vi "Init Rx - UDP Connection.vi"(8 "error in (no error)":errorcluster, 11 "Rx Loop Data in":T1) -> (0 "error out":errorcluster, 3 "Rx Loop Data out":T1)   [LabVIEW 2019, in "UDP-Custom-Device Engine.lvlib"]
uses:
  UDP-Custom-Device Engine.lvlib
  Types/Engine - Rx Loop Data.ctl
  <vilib>/NI VeriStand/VeriStand Data/Byte Buffer/Byte Buffer.lvclass
  Types/Engine - General Resources.ctl
  <vilib>/NI VeriStand/VeriStand Data/Typedefs/Typedefs.Data Types.ctl
  Shared/Types/Shared - Duplex Settings.ctl
  Shared/Types/Shared - Header Details.ctl
  Types/Engine - Data Conversion Config.ctl
  <vilib>/NI VeriStand/VeriStand Data/Byte Buffer/Byte Buffer.Mapping.ctl
  Types/Engine - Rx Runtime Resources.ctl
  Types/Engine - Execution Config.ctl
  Shared/Types/Shared - Thread Management.ctl
  Types/Engine - Rx New Data Options Support.ctl
  Shared/Types/Shared - New Data Options.ctl
  Types/Engine - Rx Channel Refs.ctl
  <vilib>/NI/NIVS Inline Async API/_Data Access Engine/Data Access Engine/Types/Write.DVR.ctl
  <vilib>/NI/NIVS Inline Async API/_Data Access Engine/Access Type Classes/Write/Write.lvclass
  Types/Engine - Debug Resources.ctl
  <vilib>/Utility/tcp.llb/UDP Multicast Read-Only Open.vi
  <vilib>/NI/NIVS Inline Async API/_Data Access Engine/Data Access Engine/Data Access Engine.lvclass
  <vilib>/NI VeriStand/VeriStand Data/VeriStand Data.lvlib
  Shared/UDP-Custom-Device Shared.lvlib
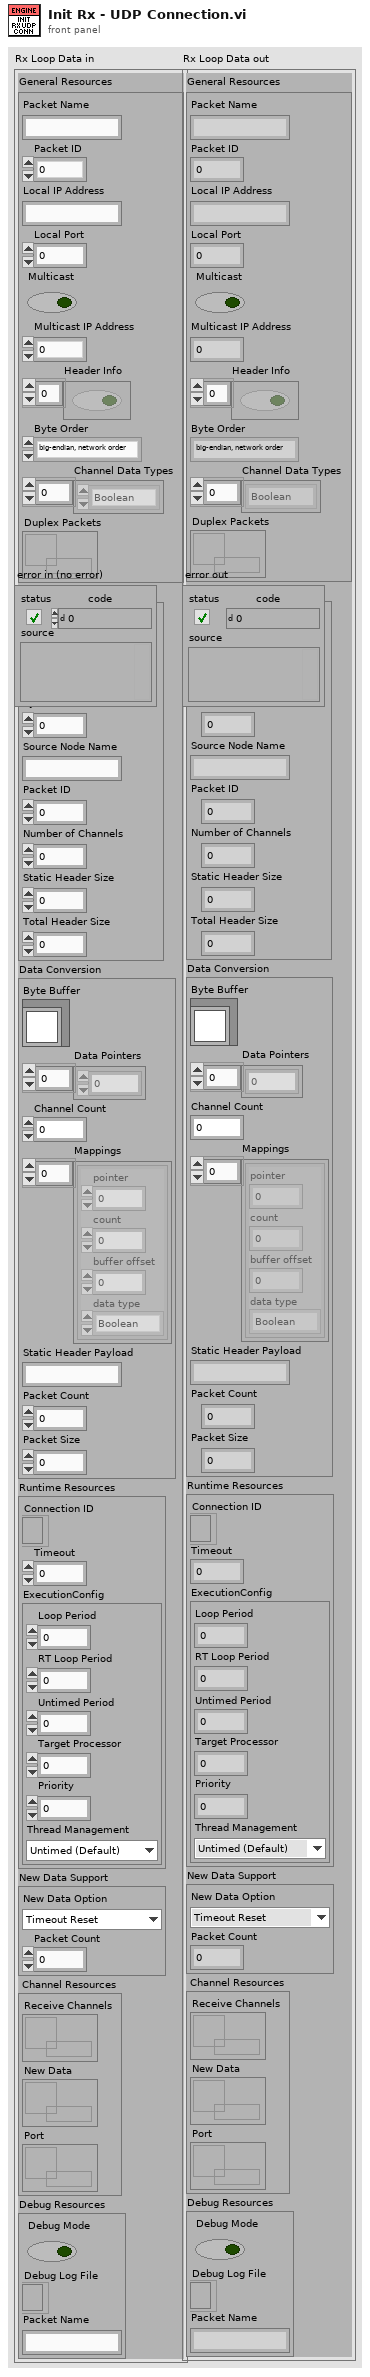
[diagram p1: front panel]
types:
  T1 = typedef "UDP-Custom-Device Engine.lvlib/Engine - Rx Loop Data.ctl" = cluster{"General Resources":T2, "Header Details":T4, "Data Conversion":T5, "Runtime Resources":T7, "New Data Support":T10, "Channel Resources":T12, "Debug Resources":T14}
  T2 = typedef "UDP-Custom-Device Engine.lvlib/Engine - General Resources.ctl" = cluster{"Packet Name":string, "Packet ID":i32, "Local IP Address":string, "Local Port":i32, "Multicast":bool, "Multicast IP Address":u32, "Header Info":bool[], "Byte Order":enum16{"big-endian, network order", "native, host order", "little-endian"}, "Channel Data Types":T3[], "Duplex Packets":refnum<data-value>}
  T3 = typedef "VeriStand Data.lvlib/Typedefs.Data Types.ctl" = enum16{"Boolean", "Single", "Double", "I8", "I16", "I32", "I64", "U8", "U16", "U32", "U64"}
  T4 = typedef "UDP-Custom-Device Shared.lvlib/Shared - Header Details.ctl" = cluster{"Packet Size":u16, "Protocol Revision":u8, "System Definition Version":u64, "Source Node Name":string, "Packet ID":u32, "Number of Channels":u32, "Static Header Size":u16, "Total Header Size":u16}
  T5 = typedef "UDP-Custom-Device Engine.lvlib/Engine - Data Conversion Config.ctl" = cluster{"Byte Buffer":refnum<class "Byte Buffer.lvclass">, "Data Pointers":u64[], "Channel Count":i32, "Mappings":T6[], "Static Header Payload":string, "Packet Count":dbl, "Packet Size":i32}
  T6 = typedef "VeriStand Data.lvlib/Byte Buffer.lvclass/Byte Buffer.Mapping.ctl" = cluster{"pointer":u64, "count":i64, "buffer offset":u64, "data type":T3}
  T7 = typedef "UDP-Custom-Device Engine.lvlib/Engine - Rx Runtime Resources.ctl" = cluster{"Connection ID":refnum<k16>, "Timeout":i32, "ExecutionConfig":T8}
  T8 = typedef "UDP-Custom-Device Engine.lvlib/Engine - Execution Config.ctl" = cluster{"Loop Period":i64, "RT Loop Period":i64, "Untimed Period":u32, "Target Processor":i32, "Priority":i32, "Thread Management":T9}
  T9 = typedef "UDP-Custom-Device Shared.lvlib/Shared - Thread Management.ctl" = enum16{"Untimed (Default)", "Timed (High Priority)"}
  T10 = typedef "UDP-Custom-Device Engine.lvlib/Engine - Rx New Data Options Support.ctl" = cluster{"New Data Option":T11, "Packet Count":dbl}
  T11 = typedef "UDP-Custom-Device Shared.lvlib/Shared - New Data Options.ctl" = enum16{"Timeout Reset", "Counter"}
  T12 = typedef "UDP-Custom-Device Engine.lvlib/Engine - Rx Channel Refs.ctl" = cluster{"Receive Channels":T13, "New Data":T13, "Port":T13}
  T13 = typedef "Data Access Engine.lvlib/Data Access Engine.lvclass/Write.DVR.ctl" = refnum<data-value>
  T14 = typedef "UDP-Custom-Device Engine.lvlib/Engine - Debug Resources.ctl" = cluster{"Debug Mode":bool, "Debug Log File":refnum<file>, "Packet Name":string}
  T15 = typedef "UDP-Custom-Device Shared.lvlib/Shared - Duplex Settings.ctl" = cluster{"Transmit Packet ID":i32, "Receive Packet ID":i32, "Multicast":bool, "Multicast Address":string, "IP Address":string, "Port":u16, "TTL":u16, "Duplex Connection":refnum<k16>}
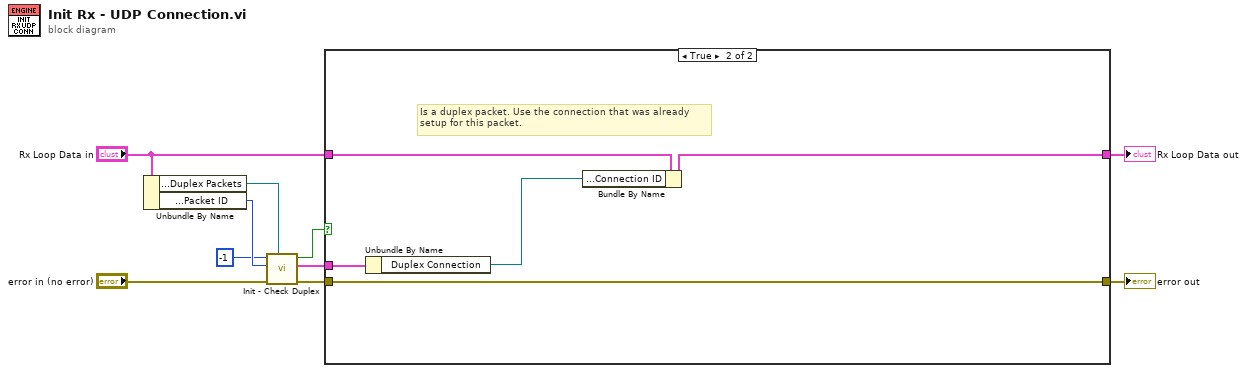
[diagram p0: block diagram]
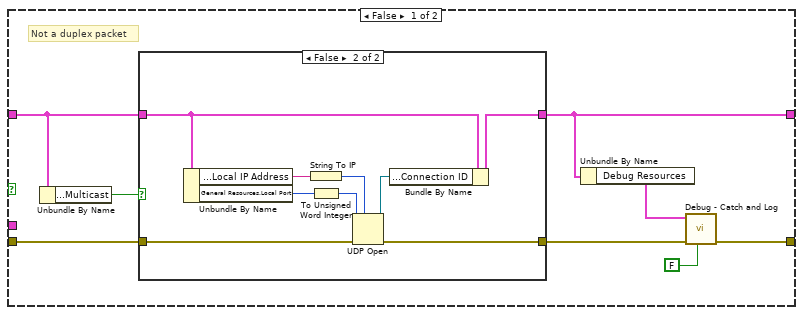
[diagram p2: hidden frame]
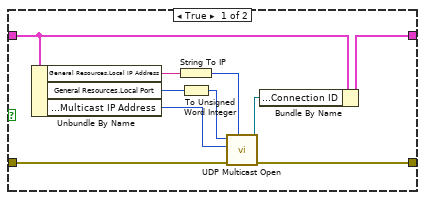
[diagram p3: hidden frame]
diagram:
  n1 = Unbundle By Name("Rx Loop Data in") -> ("General Resources.Duplex Packets"=w7:refnum<data-value>, "General Resources.Packet ID"=w6:i32)
  n2 = call "Init - Check Duplex.vi"("Duplex Packets"=w7, "error in (no error)"="error in (no error)", "Receive Packet ID"=w6, "Transmit Packet ID"=-1) -> ("error out"=w4:errorcluster, "Duplex Settings"=w3:T15, "Is Duplex?"=w2:bool)  [unwired: 5 in]
  n3 = case shown="True" w2 {
    tunnel: "Rx Loop Data in" -> [w17 w40]
    tunnel: w4 -> [w16 w41]
    tunnel: [w12 w41] -> w10
    tunnel: [w13 w38] -> w9
    tunnel: w3 -> [_ w42]
    frame False {
      # "Not a duplex packet"
      # "Not a duplex packet"
      n4 = Unbundle By Name(w17) -> ("General Resources.Multicast"=w18:bool)
      n5 = case shown="False" w18 {
        tunnel: w17 -> [w26 w32]
        tunnel: [w25 w31] -> w13
        tunnel: w16 -> [w20 w30]
        tunnel: [w19 w29] -> w11
        frame True {
          n6 = Unbundle By Name(w26) -> ("General Resources.Local IP Address"=w28:string, "General Resources.Local Port"=w27:i32, "General Resources.Multicast IP Address"=w22:u32)
          n7 = String To IP(1:w28) -> (0:w24:u32)
          n8 = To Unsigned Word Integer(number=w27) -> (unsigned 16bit integer=w23:u16)
          n9 = call-poly <vilib>:"UDP Multicast Open.vi"("net address"=w24, "error in (no error)"=w20, "multicast addr"=w22, "port"=w23) -> ("error out"=w19:errorcluster, "connection ID"=w21:refnum<k16>)  [unwired: 5 in, 1 out]
          n10 = Bundle By Name(cluster=w26, "Runtime Resources.Connection ID"=w21) -> (w25:T1)
        }
        frame False {
          n11 = Unbundle By Name(w32) -> ("General Resources.Local IP Address"=w34:string, "General Resources.Local Port"=w33:i32)
          n12 = String To IP(1:w34) -> (0:w35:u32)
          n13 = To Unsigned Word Integer(number=w33) -> (unsigned 16bit integer=w36:u16)
          n14 = UDP Open(7:w35, 8:w30, 11:w36) -> (port=w37:refnum<k16>, 0:w29:errorcluster)  [unwired: 2 in, 1 out]
          n15 = Bundle By Name(cluster=w32, "Runtime Resources.Connection ID"=w37) -> (w31:T1)
        }
      }
      n16 = Unbundle By Name(w13) -> ("Debug Resources"=w14:T14)
      n17 = call "Debug - Catch and Log.vi"("Clear Error?"=FALSE, "error in (no error)"=w11, "Debug Resources"=w14) -> ("error out"=w12:errorcluster)  [unwired: 8 in]
    }
    frame True {
      # "Is a duplex packet. Use the connection that was already\nsetup for this packet."
      n18 = Unbundle By Name(w42) -> ("Duplex Connection"=w39:refnum<k16>)
      n19 = Bundle By Name(cluster=w40, "Runtime Resources.Connection ID"=w39) -> (w38:T1)
    }
  }
  "Rx Loop Data out" <- w9
  "error out" <- w10
